vi "Non Supported Function Dialog.vi"(6 "Update Setting:":T1, 8 "error in":errorcluster, 10 "Supported?":bool, 11 "Camera in":refnum<class "Camera.lvclass">) -> (0 "error out":errorcluster, 3 "Camera out":refnum<class "Camera.lvclass">)   [LabVIEW 2018, in "Camera.lvlib" / "Camera.lvclass"]
uses:
  Camera.lvclass
  Custom Controls/Camera Setting.ctl
  Camera.lvclass/Camera.ctl
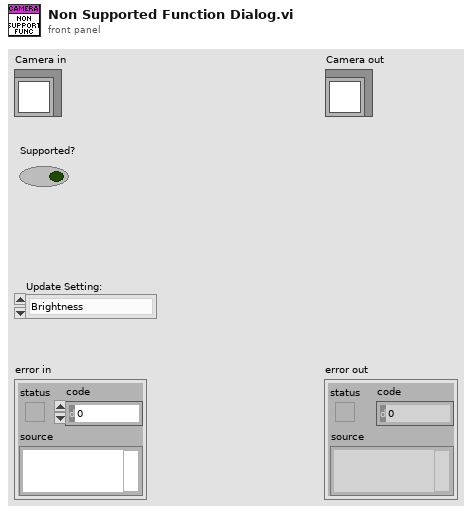
[diagram p1: front panel]
types:
  T1 = typedef "Camera.lvlib/Camera.lvclass/Camera Setting.ctl" = enum16{"Brightness", "Rotation", "Contrast", "Exposure", "Frame Rate", "Gain", "Gamma", "Image Resolution", "Sharpness"}
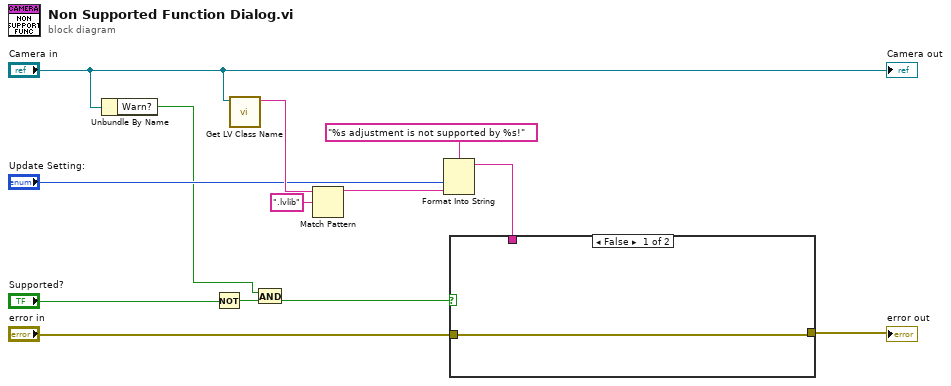
[diagram p0: block diagram]
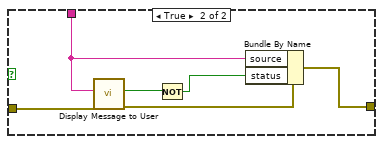
[diagram p2: hidden frame]
diagram:
  n1 = Unbundle By Name("Camera in") -> ("Warn?"=w1:bool)
  n2 = Not(x="Supported?") -> (.not. x?=w4:bool)
  n3 = call <vilib>:"Get LV Class Name.vi"("object"="Camera in") -> ("class name"=w10:string)  [unwired: 9 in, 1 out]
  n4 = And(x=w1, y=w4) -> (x .and. y?=w2:bool)
  n5 = Match Pattern(string=w10, regular expression=".lvlib") -> (before substring=w11:string)  [unwired: 1 in, 3 out]
  n6 = Format Into String(format string="%s adjustment is not supported by %s!", "Update Setting:", w11) -> (resulting string=w13:string)  [unwired: 2 in, 1 out]
  n7 = case shown="False" w2 {
    tunnel: w13 -> [_ w20]
    tunnel: [w14 w17] -> w12
    tunnel: "error in" -> [w14 w16]
    frame False {
    }
    frame True {
      n8 = call "Display Message to User"("error in (no error)"=w16, "Message"=w20) -> ("error out"=w15:errorcluster, "OK"=w18:bool)  [unwired: 8 in]
      n9 = Not(x=w18) -> (.not. x?=w19:bool)
      n10 = Bundle By Name(cluster=w15, "source"=w20, "status"=w19) -> (w17:errorcluster)
    }
  }
  "error out" <- w12
  "Camera out" <- "Camera in"
